vi "复制模板路径.vi"(8 "错误输入":errorcluster, 11 "名称前缀":string) -> (0 "错误输出":errorcluster, 3 "新路径":path)   [LabVIEW 2020]
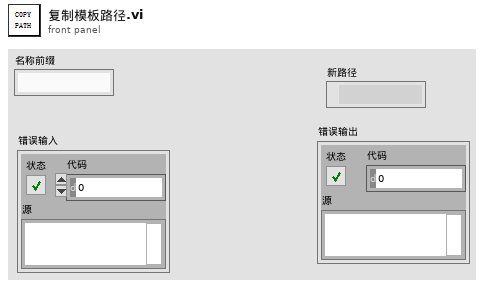
[diagram p1: front panel]
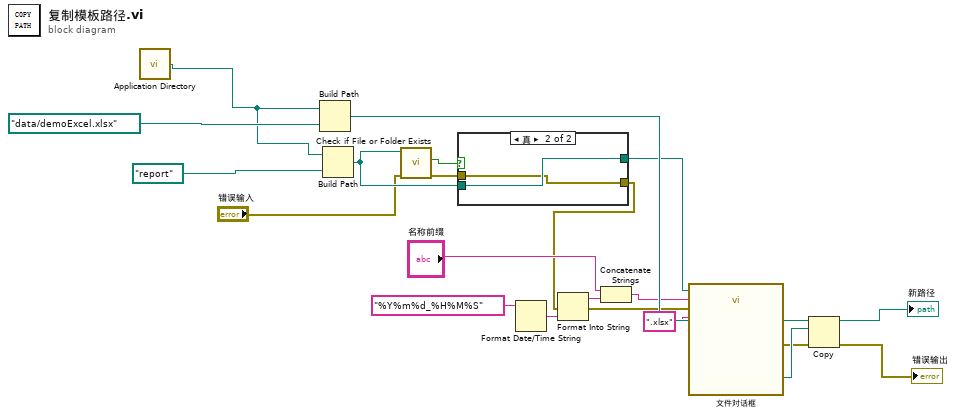
[diagram p0: block diagram]
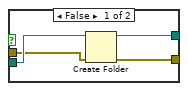
[diagram p2: hidden frame]
diagram:
  n1 = call <vilib>:"Application Directory.vi"() -> ("Application Directory"=w7:path)
  n2 = Build Path(base path=w7, name or relative path=path "data/demoExcel.xlsx" ("名称或相对路径")) -> (appended path=w21:path)
  n3 = Build Path(base path=w7, name or relative path=path "report" ("名称或相对路径")) -> (appended path=w5:path)
  n4 = call <vilib>:"Check if File or Folder Exists.vi"("error in (no error)"="错误输入", "path"=w5) -> ("error out"=w4:errorcluster, "file or folder exists?"=w6:bool)  [unwired: 7 in, 1 out]
  n5 = case shown="真" w6 {
    tunnel: w5 -> [w25 w27]
    tunnel: [w23 w27] -> w3
    tunnel: w4 -> [w24 w26]
    tunnel: [w22 w26] -> w1
    frame False {
      n6 = Create Folder(path (use dialog)=w25, error in=w24) -> (created path=w23:path, error out=w22:errorcluster)  [unwired: 1 in, 1 out]
    }
    frame True {
    }
  }
  n7 = Format Date/Time String(time format string (%c)="%Y%m%d_%H%M%S" ("时间格式字符串(%c)")) -> (date/time string=w16:string)  [unwired: 2 in]
  n8 = Format Into String(error in=w1, w16) -> (resulting string=w15:string, error out=w13:errorcluster)  [unwired: 2 in]
  n9 = Concatenate Strings("名称前缀", w15) -> (w14:string)
  n10 = call "文件对话框"("start path"=w3, "default name"=w14, "error in"=w13, "pattern (all files)"=".xlsx") -> ("selected path"=w20:path, "error out"=w19:errorcluster)  [unwired: 8 in, 2 out]
  n11 = Copy(8:w19, 10:w20, 11:w21) -> (0:→"错误输出":errorcluster, 3:→"新路径":path)  [unwired: 2 in, 1 out]
